vi "Day_3.vi"() -> ()   [LabVIEW 2018]
uses:
  Global 1.vi
  <vilib>/measure/NI_MABase.lvlib
panel:
  in  "Down":bool
  out "current time":timestamp
  in  "Stoppp":bool
  in  "Change":bool
  out "Numeric 13":dbl
  in  "Numeric 12":dbl
  in  "Numeric 9":dbl
  in  "Div":bool
  in  "Add":bool
  in  "Sub":bool
  in  "Mul":bool
  in  "Calculate":bool
  out "Waveform Chart":waveform(dbl)(graph)
  in  "Array 2":cluster{"Numeric 10":dbl, "Boolean":bool}[](array[cluster])
  in  "Array":dbl[][](array[numeric])
  in  "sampling info":cluster{"Fs":dbl, "#s":dbl}={"Fs"=1000.0, "#s"=1000.0} {"Fs" format="%.2p"}
  out "String":string
  in  "Numeric 8":i16
  out "x/y":dbl
  out "x*y":dbl
  out "x-y":dbl
  in  "Numeric 11":dbl
  in  "Numeric 10":dbl
  out "x+y":dbl
  in  "Enum":enum16{"Add", "Sub", "Mul", "Div"}(ring)
  out "Boolean 3":bool
  in  "Numeric 7":dbl
  in  "Numeric 6":dbl
  in  "Numeric 5":dbl
  in  "Numeric 4":dbl
  out "Boolean 2":bool
  in  "stop":bool
  in  "Numeric 3":dbl
  out "Boolean":bool
  in  "Numeric 2":dbl
  in  "Numeric":dbl
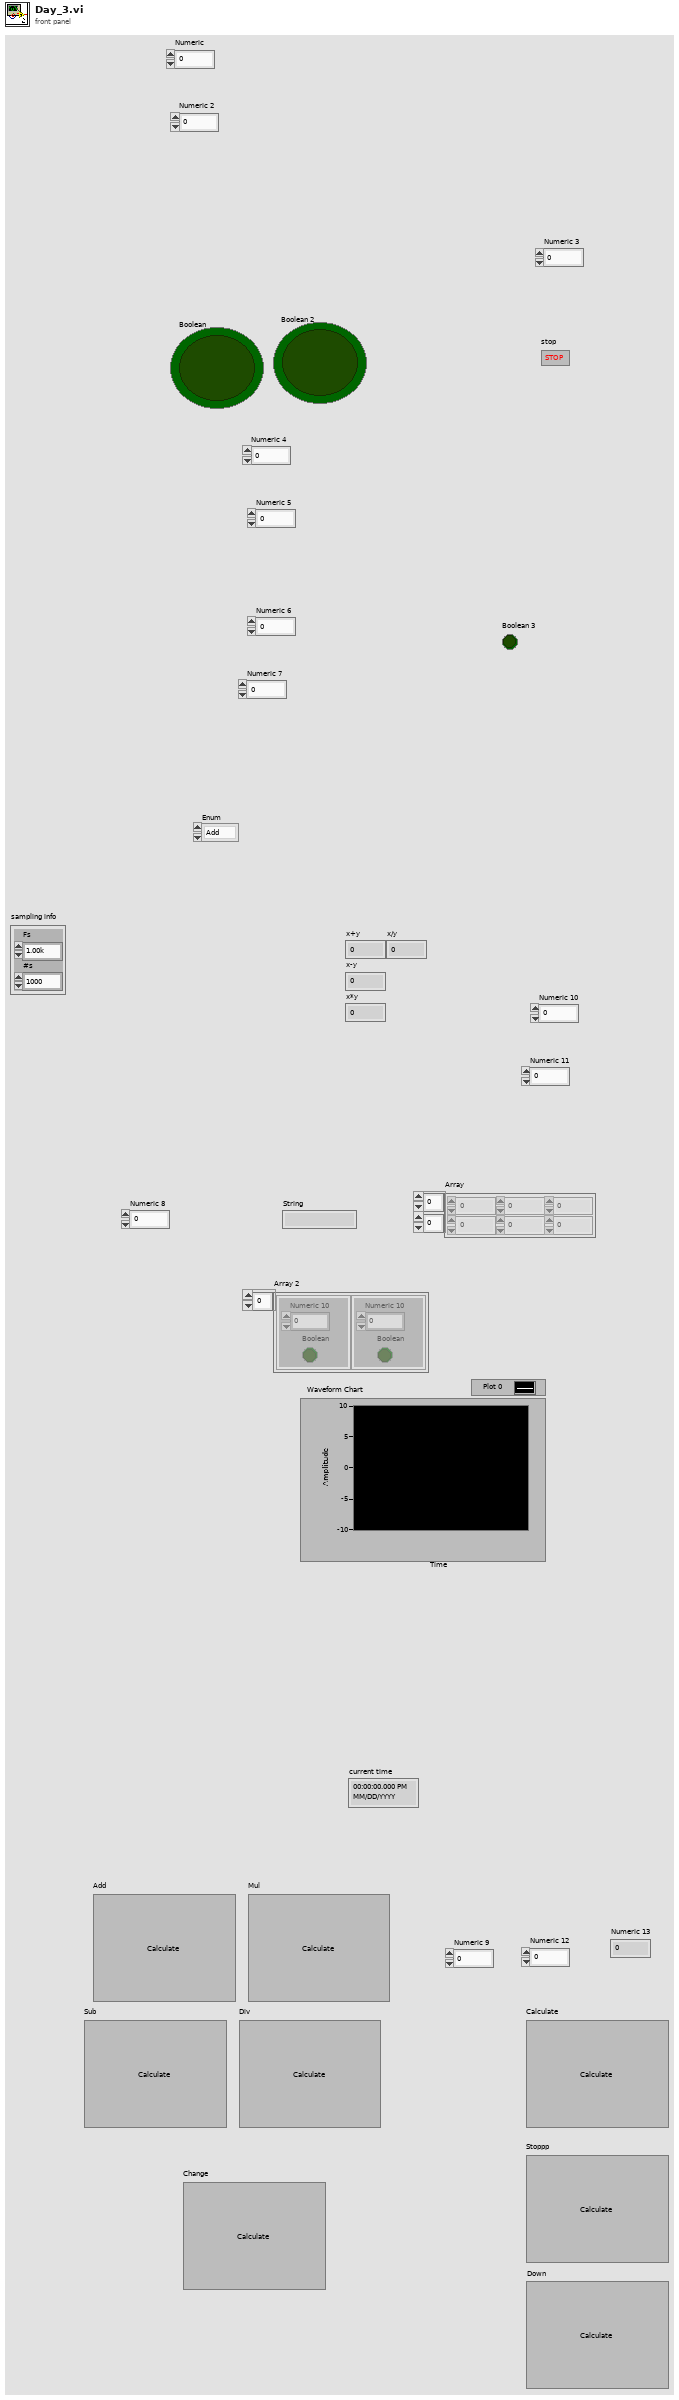
[diagram p1: front panel]
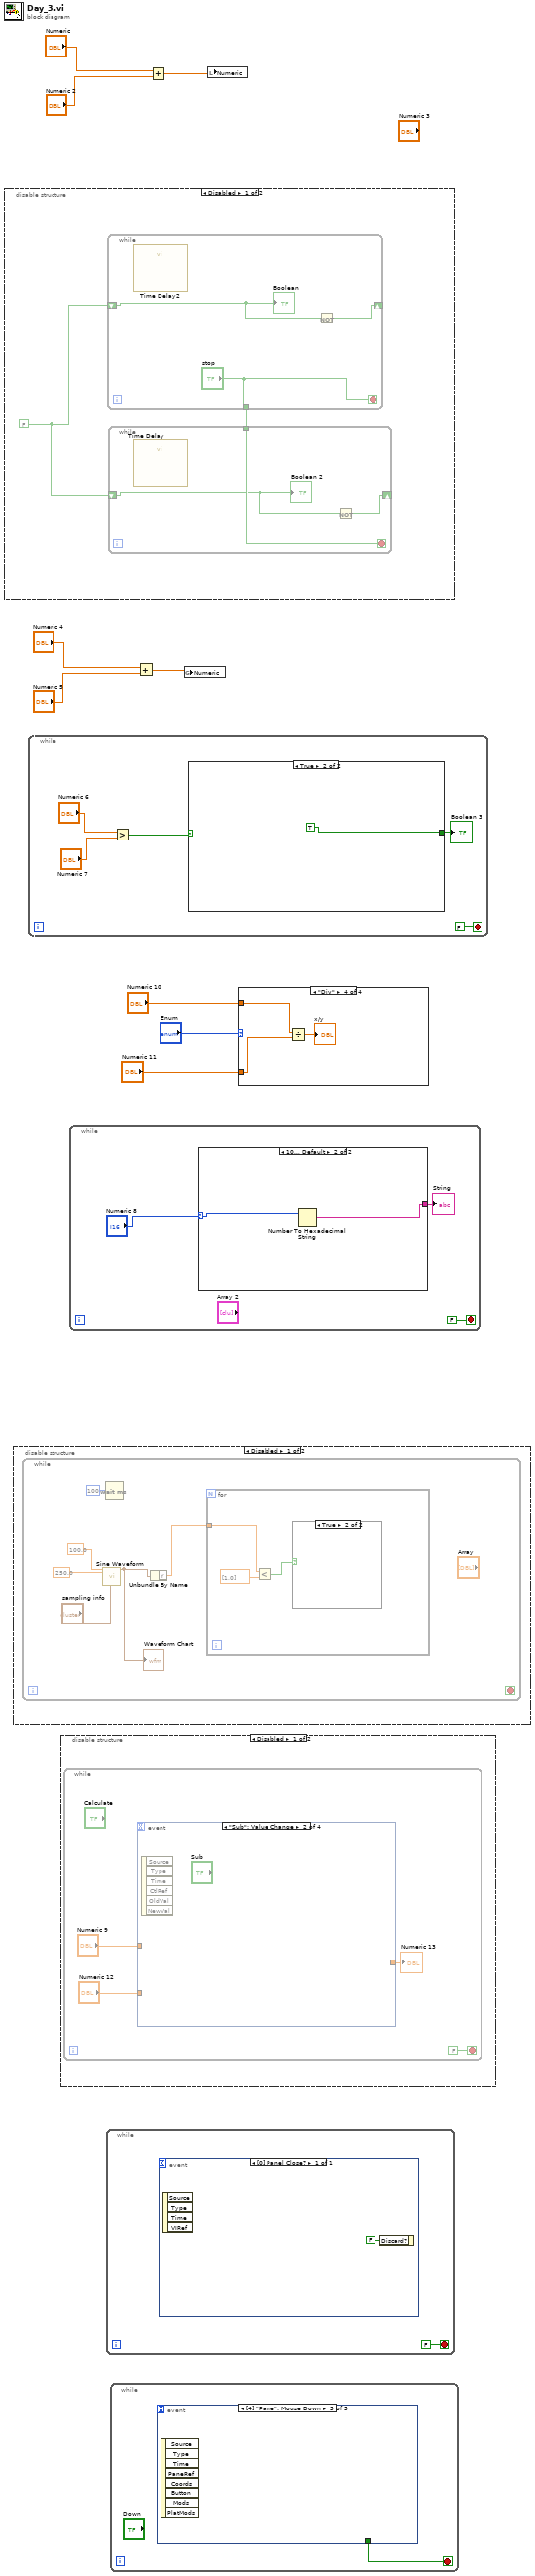
[diagram p0: block diagram]
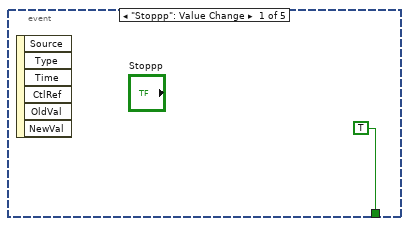
[diagram p2: hidden frame]
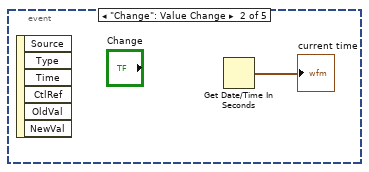
[diagram p3: hidden frame]
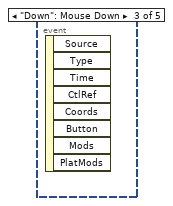
[diagram p4: hidden frame]
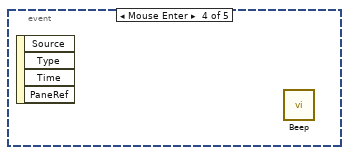
[diagram p5: hidden frame]
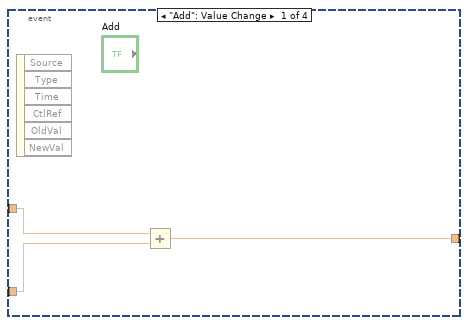
[diagram p6: hidden frame]
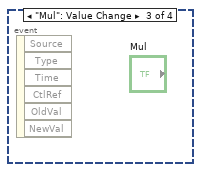
[diagram p7: hidden frame]
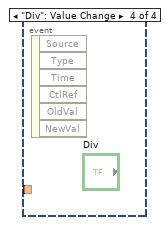
[diagram p8: hidden frame]
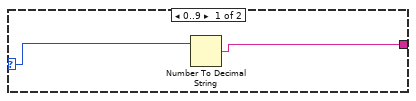
[diagram p12: hidden frame]
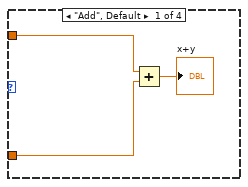
[diagram p13: hidden frame]
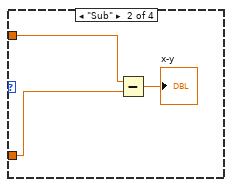
[diagram p14: hidden frame]
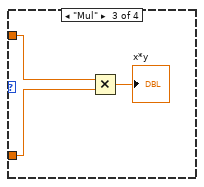
[diagram p15: hidden frame]
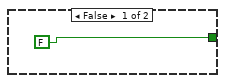
[diagram p16: hidden frame]
diagram:
  n1 = disable-structure shown="Disabled" {
    frame Disabled {
      w10 = FALSE
      n2 = while {
        shift-right: [w16] -> _
        shift-left: w10 -> [w17]
        tunnel: ["stop"] -> w11
        stop <- "stop" stop-if-true
        n3 = call "Time Delay2"() -> ()  [unwired: 11 in, 1 out]
        n4 = Not(x=w17) -> (.not. x?=w16:bool)
        "Boolean" <- w17
      }
      n5 = while {
        shift-right: [w12] -> _
        shift-left: w10 -> [w13]
        tunnel: w11 -> [w14]
        stop <- w14 stop-if-true
        n6 = call "Time Delay"() -> ()  [unwired: 11 in, 1 out]
        n7 = Not(x=w13) -> (.not. x?=w12:bool)
        "Boolean 2" <- w13
      }
    }
    frame Enabled {
    }
  }
  n8 = disable-structure shown="Disabled" {
    frame Disabled {
      n9 = while {
        stop <- _ stop-if-true
        n10 = call <vilib>:"Sine Waveform.vi"("sampling info"="sampling info", "amplitude"=250.0, "frequency"=100.0) -> ("signal out"=w19:waveform(dbl))  [unwired: 7 in, 1 out]
        "Waveform Chart" <- w19
        n11 = Wait (ms)(milliseconds to wait=u32 100) -> ()  [unwired: 1 out]
        n12 = Unbundle By Name(w19) -> ("Y"=w21:dbl[])
        n13 = for {
          tunnel: w21 -> [w26]
          n14 = Less?(x=w26, y=dbl[] [1.0]) -> (x < y?=w24:bool[])
          n15 = case shown="True" w24 {
            frame False {
            }
            frame True {
            }
          }
        }
      }
    }
    frame Enabled {
    }
  }
  n16 = while {
    stop <- FALSE stop-if-true
    n17 = Greater?(x="Numeric 6", y="Numeric 7") -> (0:w29:bool)
    n18 = case shown="True" w29 {
      tunnel: [FALSE ("Boolean 4") TRUE ("Boolean")] -> w27
      frame False {
      }
      frame True {
      }
    }
    "Boolean 3" <- w27
  }
  n19 = disable-structure shown="Disabled" {
    frame Disabled {
      n20 = while {
        stop <- FALSE stop-if-true
        n21 = event shown="[1] \"Sub\": Value Change" {
          selector: _ -> [_ _ _ _]
          dyn-events: _ -> [_ _ _ _]
          timeout: _ -> [_ _ _ _]
          tunnel: "Numeric 9" -> [w40 _ _ _]
          tunnel: "Numeric 12" -> [w39 _ _ _]
          tunnel: [w38 _ _ _] -> w34
          event "Add": Value Change {
            n22 = event-data() -> ()  [unwired: 1 in, 6 out]
            n23 = Add(x=w40, y=w39) -> (x+y=w38:dbl)
          }
          event "Sub": Value Change {
            n24 = event-data() -> ()  [unwired: 1 in, 6 out]
          }
          event "Mul": Value Change {
            n25 = event-data() -> ()  [unwired: 1 in, 6 out]
          }
          event "Div": Value Change {
            n26 = event-data() -> ()  [unwired: 1 in, 6 out]
          }
        }
        "Numeric 13" <- w34
      }
    }
    frame Enabled {
    }
  }
  n27 = while {
    stop <- FALSE stop-if-true
    n28 = case shown="10.., Default" "Numeric 8" {
      selector: "Numeric 8" -> [w45 w47]
      tunnel: [w44 w46] -> w41
      frame 0..9 {
        n29 = Number To Decimal String(number=w45) -> (decimal integer string=w44:string)  [unwired: 1 in]
      }
      frame 10.., Default {
        n30 = Number To Hexadecimal String(2:w47) -> (0:w46:string)  [unwired: 1 in]
      }
    }
    "String" <- w41
  }
  n31 = while {
    stop <- FALSE stop-if-true
    n32 = event shown="[0] Panel Close?" {
      selector: _ -> [_]
      dyn-events: _ -> [_]
      timeout: _ -> [_]
      event Panel Close? {
        n33 = event-data() -> ()  [unwired: 1 in, 4 out]
        n34 = event-data("Discard?"=FALSE) -> ()  [unwired: 1 in, 1 out]
      }
    }
  }
  n35 = while {
    stop <- w50 stop-if-true
    n36 = event shown="[4] \"Pane\": Mouse Down" {
      selector: _ -> [_ _ _ _ _]
      dyn-events: _ -> [_ _ _ _ _]
      timeout: _ -> [_ _ _ _ _]
      tunnel: [TRUE _ _ _ _] -> w50
      event "Stoppp": Value Change {
        n37 = event-data() -> ()  [unwired: 1 in, 6 out]
      }
      event "Change": Value Change {
        n38 = event-data() -> ()  [unwired: 1 in, 6 out]
        n39 = Get Date/Time In Seconds() -> (seconds since 1Jan1904=→"current time":timestamp)
      }
      event "Down": Mouse Down {
        n40 = event-data() -> ()  [unwired: 1 in, 8 out]
      }
      event Mouse Enter {
        n41 = event-data() -> ()  [unwired: 1 in, 4 out]
        n42 = call <vilib>:"Beep.vi"() -> ()  [unwired: 12 in]
      }
      event Mouse Down {
        n43 = event-data() -> ()  [unwired: 1 in, 8 out]
      }
    }
  }
  n44 = Add(x="Numeric 4", y="Numeric 5") -> (x+y=w4:dbl)
  n45 = Add(x="Numeric", y="Numeric 2") -> (x+y=w7:dbl)
  n46 = global write "Global 1.vi" "Numeric"(w4) -> ()
  n47 = local write "Numeric"(w7) -> ()
  n48 = case shown="\"Div\"" "Enum" {
    tunnel: "Numeric 10" -> [w54 w58 w61 w64]
    tunnel: "Numeric 11" -> [w53 w57 w60 w63]
    frame "Add", Default {
      n49 = Add(x=w54, y=w53) -> (x+y=→"x+y":dbl)
    }
    frame "Sub" {
      n50 = Subtract(x=w58, y=w57) -> (x-y=→"x-y":dbl)
    }
    frame "Mul" {
      n51 = Multiply(x=w61, y=w60) -> (x*y=→"x*y":dbl)
    }
    frame "Div" {
      n52 = Divide(x=w64, y=w63) -> (x/y=→"x/y":dbl)
    }
  }
